vi "One Scan action.vi"(4 "Action":i32, 5 "OSC Configuration in":T3(array[cluster]), 6 "index":i32, 7 "Comments in":string, 9 "Sorted scan parameters":T2(array[cluster]), 10 "Sorted scan control":T1(array[cluster]), 11 "Additional action (indexing priority)":u16[](array[numeric])) -> (1 "Comments out":string, 2 "OSC Configuration out":T3(array[cluster]), 3 "Stop?":bool)   [LabVIEW 2013]
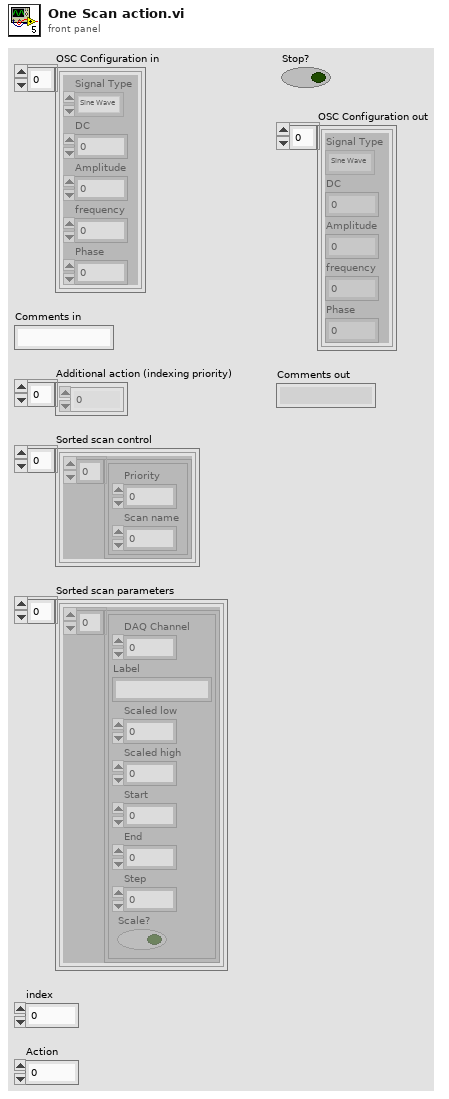
[diagram p1: front panel]
types:
  T1 = cluster{cluster{"Priority":u16, "Scan name":u16}[]}[]
  T2 = cluster{cluster{"DAQ Channel":i32, "Label":string, "Scaled low":dbl, "Scaled high":dbl, "Start":dbl, "End":dbl, "Step":dbl, "Scale?":bool}[]}[]
  T3 = cluster{"Signal Type":enum16{"Sine Wave", "Triangle Wave", "Square Wave", "Sawtooth Wave"}, "DC":dbl, "Amplitude":dbl, "frequency":dbl, "Phase":dbl}[]
  T4 = cluster{cluster{"Priority":u16, "Scan name":u16}[]}
  T5 = cluster{cluster{"DAQ Channel":i32, "Label":string, "Scaled low":dbl, "Scaled high":dbl, "Start":dbl, "End":dbl, "Step":dbl, "Scale?":bool}[]}
  T6 = cluster{"DAQ Channel":i32, "Label":string, "Scaled low":dbl, "Scaled high":dbl, "Start":dbl, "End":dbl, "Step":dbl, "Scale?":bool}[]
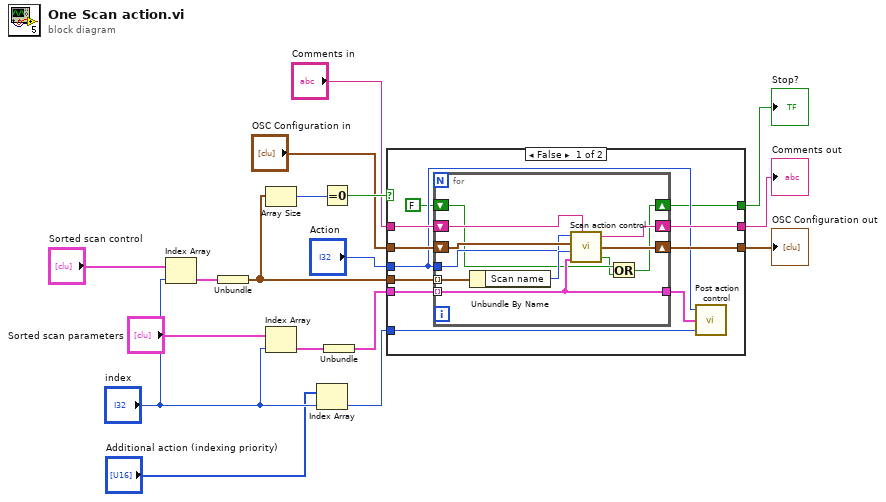
[diagram p0: block diagram]
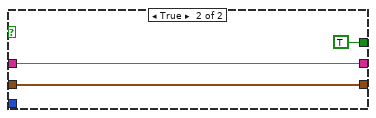
[diagram p2: hidden frame]
diagram:
  n1 = Index Array(array="Sorted scan control", index="index") -> (element=w3:T4)
  n2 = Unbundle(w3) -> (w11:cluster{"Priority":u16, "Scan name":u16}[])
  n3 = Array Size(array=w11) -> (size(s)=w15:i32)
  n4 = Index Array(array="Sorted scan parameters", index="index") -> (element=w4:T5)
  n5 = Index Array(array="Additional action (indexing priority)", index="index") -> (element=w14:u16)
  n6 = Equal To 0?(x=w15) -> (x = 0?=w16:bool)
  n7 = Unbundle(w4) -> (w5:T6)
  n8 = case shown="False" w16 {
    tunnel: w5 -> [w28 _]
    tunnel: "OSC Configuration in" -> [w27 w42]
    tunnel: "Comments in" -> [w26 w41]
    tunnel: [w25 w42] -> w8
    tunnel: [w24 w41] -> w9
    tunnel: [w18 TRUE ("Stop?")] -> w10
    tunnel: w11 -> [w23 _]
    tunnel: "Action" -> [w20 _]
    tunnel: w14 -> [w21 _]
    frame False {
      n9 = for {
        tunnel: w23 -> [w39] mode=indexing
        tunnel: w28 -> [w32] mode=indexing
        tunnel: w20 -> [w33]
        shift-right: [w37] -> w25
        shift-left: w27 -> [w36]
        shift-right: [w35] -> w24
        shift-left: w26 -> [w34]
        tunnel: [w32] -> w22
        shift-right: [w29] -> w18
        shift-left: FALSE -> [w31]
        n10 = Unbundle By Name(w39) -> ("Scan name"=w38:u16)
        n11 = call "Scan action control.vi"("Index"=w33, "OSC Configuration"=w36, "Scan control"=w38, "Scan Parameters"=w32, "Comments"=w34) -> ("Comments out"=w35:string, "OSC Configuration out"=w37:T3, "Stop?"=w30:bool)
        n12 = Or(x=w31, y=w30) -> (x .or. y?=w29:bool)
      }
      n13 = call "Post action control.vi"("Action"=w21, "Scan Parameters"=w22, "Index"=w20) -> ()  [unwired: 1 out]
    }
    frame True {
    }
  }
  "Stop?" <- w10
  "Comments out" <- w9
  "OSC Configuration out" <- w8
